vi "Test Circular Buffer.vi"() -> ()   [LabVIEW 2019, in "Instrument.Lockin.lvlib" / "Instrument UI.Lockin.lvclass"]
uses:
  Instrument UI.Lockin.lvclass
  <vilib>/PRIrvin/XY Utilities/subVIs/Circular Buffer (waveforms).vi
  <vilib>/measure/NI_MABase.lvlib
  <vilib>/PRIrvin/XY Utilities/xy_utilities.lvlib
panel:
  in  "amplitude 2":dbl=1.0 format="%0.2p"
  in  "signal type 2":T1(ring)
  in  "#s":dbl
  in  "signal type":T1(ring)
  in  "amplitude":dbl=1.0 format="%0.2p"
  out "Waveform Graph":waveform(dbl)[](graph)
  in  "stop":bool
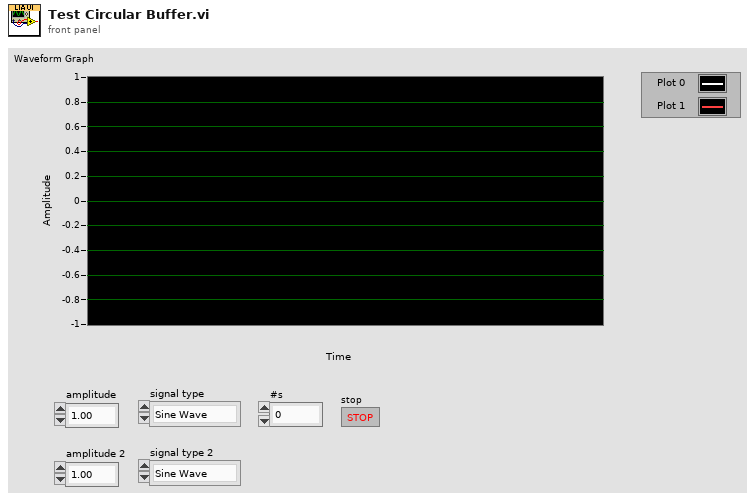
[diagram p1: front panel]
types:
  T1 = enum16{"Sine Wave", "Triangle Wave", "Square Wave", "Sawtooth Wave"}
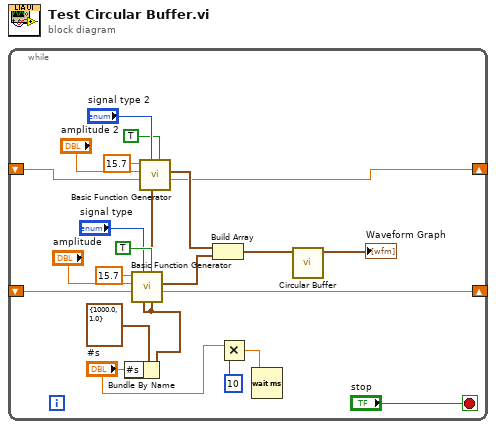
[diagram p0: block diagram]
diagram:
  n1 = while {
    shift-right: [w20] -> _
    shift-left: _ -> [w21]
    shift-right: [w4] -> _
    shift-left: _ -> [w5]
    stop <- "stop" stop-if-true
    n2 = Bundle By Name(cluster=cluster{"Fs":dbl, "#s":dbl} {"Fs"=1000.0, "#s"=1.0} ("sampling info"), "#s"="#s") -> (w3:cluster{"Fs":dbl, "#s":dbl})
    n3 = call <vilib>:"Basic Function Generator.vi"("reset signal"=TRUE, "sampling info"=w3, "signal type"="signal type", "phase"=w21, "amplitude"="amplitude", "frequency"=15.7) -> ("phase out"=w20:dbl, "signal out"=w17:waveform(dbl))  [unwired: 3 in, 1 out]
    n4 = call <vilib>:"Basic Function Generator.vi"("reset signal"=TRUE, "sampling info"=w3, "signal type"="signal type 2", "phase"=w5, "amplitude"="amplitude 2", "frequency"=15.7) -> ("phase out"=w4:dbl, "signal out"=w6:waveform(dbl))  [unwired: 3 in, 1 out]
    n5 = Build Array(w6, w17) -> (w2:waveform(dbl)[])
    n6 = Multiply(x="#s", y=u32 10 ("milliseconds to wait")) -> (x*y=w11:dbl)
    n7 = Wait (ms)(milliseconds to wait=w11) -> ()  [unwired: 1 out]
    n8 = call-poly <vilib>:"Circular Buffer.vi"("Waveform in"=w2) -> ("Waveform out"=→"Waveform Graph":waveform(dbl)[])  [unwired: 9 in, 1 out]
  }
